vi "temp-control-tuner.vi"() -> ()   [LabVIEW 2013]
uses:
  <vilib>/Analysis/polynomials.llb/Scalar Polynomial Evaluation (DBL).vi
  <vilib>/Analysis/NI_AALPro.lvlib
panel:
  in  "Output Enable":bool
  in  "pwm_rate":dbl min=0.0 max=655.35
  in  "i_limit":u8
  in  "ki":dbl min=0.0 max=65.535
  in  "kp":dbl min=0.0 max=65.535
  in  "Write Tuning":bool
  in  "Temp Setpoint (degF)":dbl=32.0 min=32.0 max=1832.0 step=1.0
  out "Array":dbl[](array[numeric])
  in  "Write Setpoint":bool
  out "Waveform Chart":T1(graph)={"[0]"=63.3344, "[1]"=32.0, "[2]"=32.0, "[3]"=32.0, "[4]"=0.0, "[5]"=0.0, "[6]"=0.0, "[7]"=0.0, "[8]"=0.0}
  in  "stop":bool
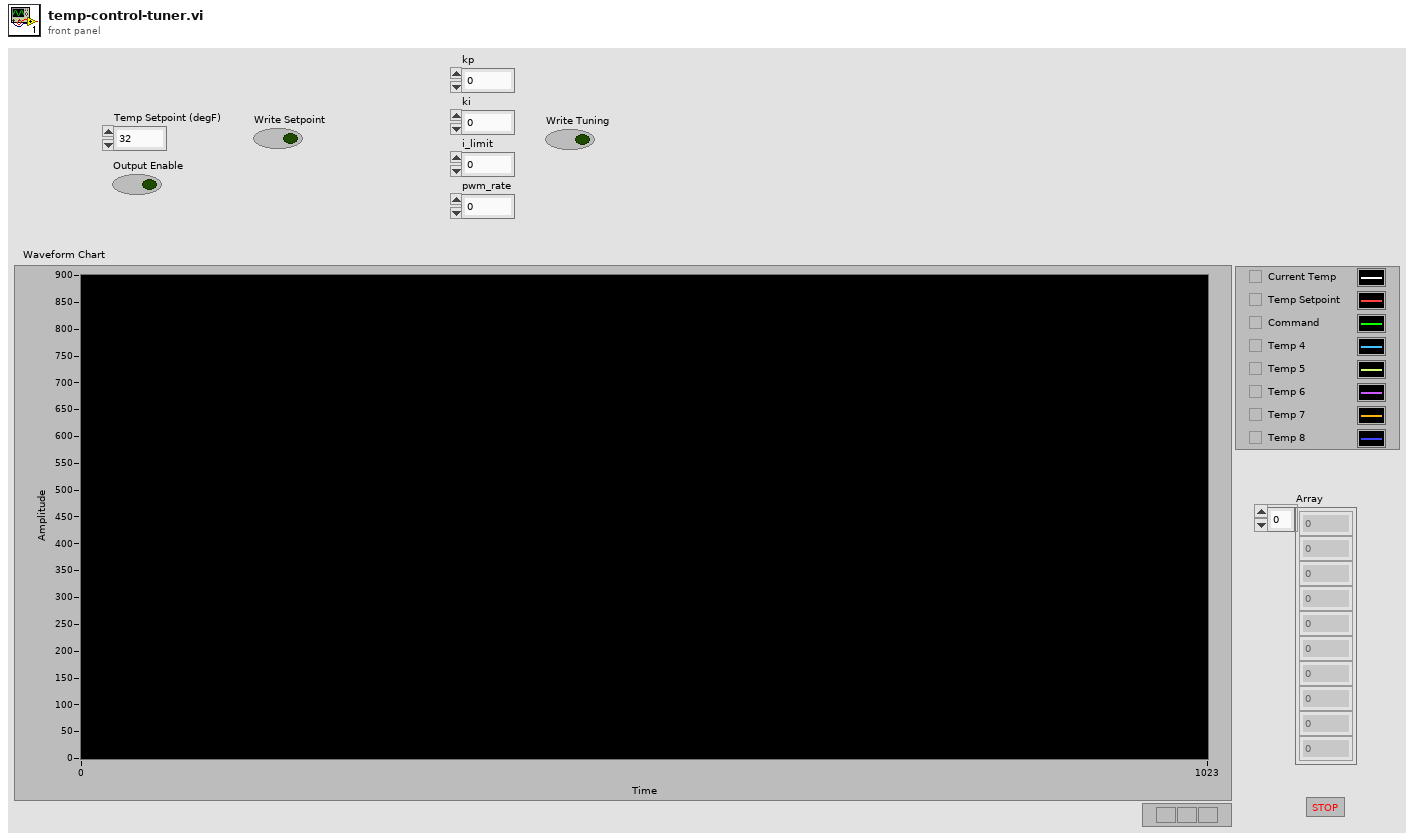
[diagram p1: front panel]
types:
  T1 = cluster{"[0]":dbl, "[1]":dbl, "[2]":dbl, "[3]":dbl, "[4]":dbl, "[5]":dbl, "[6]":dbl, "[7]":dbl, "[8]":dbl}
  T2 = enum16{"HSCAN", "MSCAN", "SWCAN", "LSFTCAN", "HSCAN2", "HSCAN3"}
  T3 = cluster{"DeviceType":i32, "Handle":i32, "NumberOfClients":i32, "SerialNumber":i32, "MaxAllowedClients":i32}[]
  T4 = cluster{"DeviceType":i32, "Handle":i32, "NumberOfClients":i32, "SerialNumber":i32, "MaxAllowedClients":i32}
  T5 = enum16{"DEVICE", "HSCAN", "MSCAN", "SWCAN", "LSFTCAN", "FORDSCP", "J1708", "JVPW", "ISO", "FIRE_HSCAN2", "FIRE_MSCAN1", "FIRE_HSCAN3", "FIRE_LIN2", "FIRE_LIN3", "FIRE_LIN4"}
  T6 = typedef "ctl spymessage.ctl" = cluster{"StatusBitField":u32, "StatusBitField2":u32, "TimeHardware":u32, "TimeHardware2":u32, "TimeSystem":u32, "TimeSystem2":u32, "TimeStampHardwareID":u8, "TimeStampHardwareID2":u8, "NetworkID":u8, "NodeID":u8, "Protocol":u8, "MessagePieceID":u8, "ColorID":u8, "NumberBytesHeader":u8, "NumberBytesData":u8, "DescriptionID":u16, "ArbIDOrHeader":u32, "Data [8]":u8[], "AckBytes [8]":u8[], "Value":sgl, "MiscData":u8}
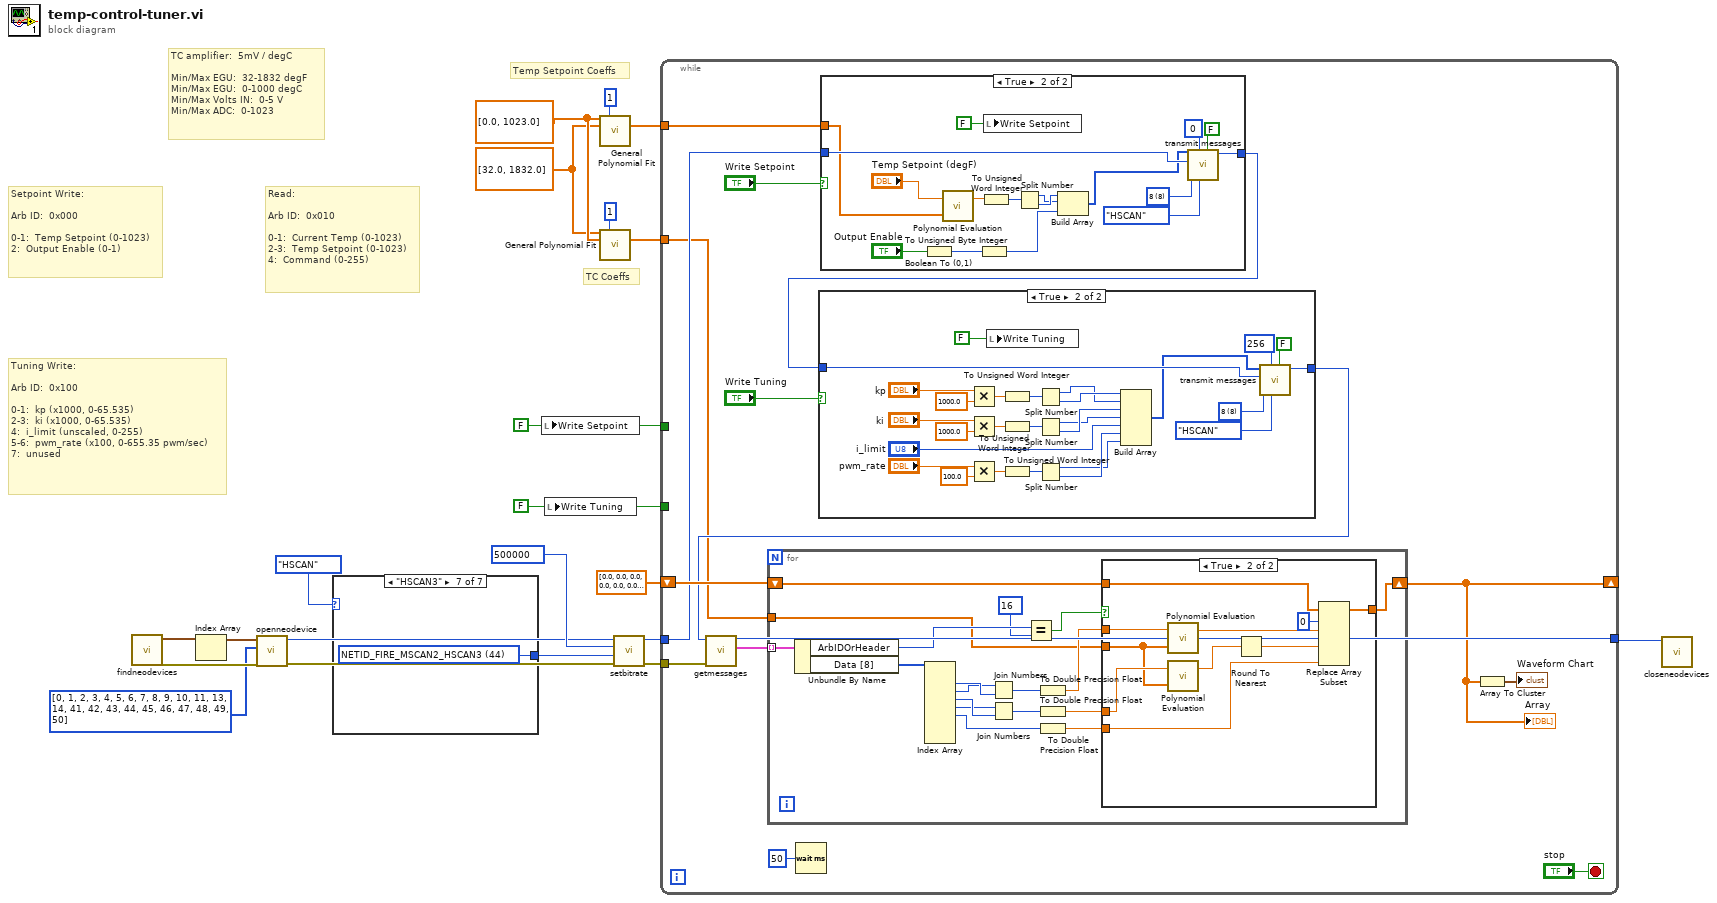
[diagram p0: block diagram]
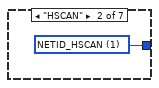
[diagram p3: hidden frame]
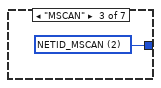
[diagram p4: hidden frame]
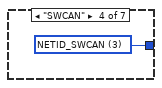
[diagram p5: hidden frame]
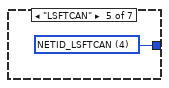
[diagram p6: hidden frame]
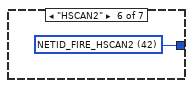
[diagram p7: hidden frame]
diagram:
  w5 = FALSE ("Send")
  w1 = dbl[] [32.0, 1832.0] ("Y")
  w2 = dbl[] [0.0, 1023.0] ("Y")
  w8 = FALSE ("Send")
  w15 = 500000 items=["20000"=20000, "33333"=33333, "50000"=50000, "62500"=62500, "83333"=83333, "100000"=100000, "125000"=125000, "250000"=250000, "500000"=500000, "800000"=800000, "1000000"=1000000] ("Bit Rate")
  w18 = i8[] [0, 1, 2, 3, 4, 5, 6, 7, 8, 9, 10, 11, 13, 14, 41, 42, 43, 44, 45, 46, 47, 48, 49, 50] items=["NETID_DEVICE"=0, "NETID_HSCAN"=1, "NETID_MSCAN"=2, "NETID_SWCAN"=3, "NETID_LSFTCAN"=4, "NETID_FORDSCP"=5, "NETID_J1708"=6, "NETID_AUX"=7, "NETID_JVPW"=8, "NETID_ISO_LIN"=9, "NETID_ISOPIC"=10, "NETID_MAIN51"=11, "NETID_SCI"=13, "NETID_ISO2"=14, "NETID_FIRE_HSCAN1"=41, "NETID_FIRE_HSCAN2"=42, "NETID_FIRE_MSCAN1"=43, "NETID_FIRE_MSCAN2_HSCAN3"=44, "NETID_FIRE_SWCAN"=45, "NETID_FIRE_LSFT"=46, "NETID_FIRE_LIN1"=47, "NETID_FIRE_LIN2"=48, "NETID_FIRE_LIN3"=49, "NETID_FIRE_LIN4"=50] ("bNetworkIDs")
  # "Temp Setpoint Coeffs"
  # "TC Coeffs"
  # "TC amplifier:  5mV / degC\n\nMin/Max EGU:  32-1832 degF\nMin/Max EGU:  0-1000 degC\nMin/Max Volts IN:  0-5 V\nMin/Max ADC:  0-1023"
  # "Read:\n\nArb ID:  0x010\n\n0-1:  Current Temp (0-1023)\n2-3:  Temp Setpoint (0-1023)\n4:  Command (0-255)"
  # "Tuning Write:\n\nArb ID:  0x100\n\n0-1:  kp (x1000, 0-65.535)\n2-3:  ki (x1000, 0-65.535)\n4:  i_limit (unscaled, 0-255)\n5-6:  pwm_rate (x100, 0-655.35 pwm/sec)\n7:  unused"
  # "Setpoint Write:\n\nArb ID:  0x000\n\n0-1:  Temp Setpoint (0-1023)\n2:  Output Enable (0-1)"
  n1 = call "findneodevices.vi"() -> ("error out"=w20:errorcluster, "NeoDevices {}"=w21:T3)  [unwired: 3 in, 7 out]
  n2 = Index Array(array=w21) -> (element=w19:T4)  [unwired: 1 in]
  n3 = call "openneodevice.vi"("error in (no error)"=w20, "bNetworkIDs"=w18, "NeoDevice{}"=w19) -> ("error out"=w12:errorcluster, "hObject"=w13:i32)  [unwired: 2 in, 5 out]
  n4 = case shown="\"HSCAN3\"" T2."HSCAN" ("CAN Channel") {
    tunnel: [_ w22 w23 w24 w25 w26 w27] -> w14
    frame Default {
    }
    frame "HSCAN" {
      w22 = i8 1 items=["NETID_DEVICE"=0, "NETID_HSCAN"=1, "NETID_MSCAN"=2, "NETID_SWCAN"=3, "NETID_LSFTCAN"=4, "NETID_FORDSCP"=5, "NETID_J1708"=6, "NETID_AUX"=7, "NETID_JVPW"=8, "NETID_ISO_LIN"=9, "NETID_ISOPIC"=10, "NETID_MAIN51"=11, "NETID_SCI"=13, "NETID_ISO2"=14, "NETID_FIRE_HSCAN1"=41, "NETID_FIRE_HSCAN2"=42, "NETID_FIRE_MSCAN1"=43, "NETID_FIRE_MSCAN2_HSCAN3"=44, "NETID_FIRE_SWCAN"=45, "NETID_FIRE_LSFT"=46, "NETID_FIRE_LIN1"=47, "NETID_FIRE_LIN2"=48, "NETID_FIRE_LIN3"=49, "NETID_FIRE_LIN4"=50] ("NetworkID")
    }
    frame "MSCAN" {
      w23 = i8 2 items=["NETID_DEVICE"=0, "NETID_HSCAN"=1, "NETID_MSCAN"=2, "NETID_SWCAN"=3, "NETID_LSFTCAN"=4, "NETID_FORDSCP"=5, "NETID_J1708"=6, "NETID_AUX"=7, "NETID_JVPW"=8, "NETID_ISO_LIN"=9, "NETID_ISOPIC"=10, "NETID_MAIN51"=11, "NETID_SCI"=13, "NETID_ISO2"=14, "NETID_FIRE_HSCAN1"=41, "NETID_FIRE_HSCAN2"=42, "NETID_FIRE_MSCAN1"=43, "NETID_FIRE_MSCAN2_HSCAN3"=44, "NETID_FIRE_SWCAN"=45, "NETID_FIRE_LSFT"=46, "NETID_FIRE_LIN1"=47, "NETID_FIRE_LIN2"=48, "NETID_FIRE_LIN3"=49, "NETID_FIRE_LIN4"=50] ("NetworkID")
    }
    frame "SWCAN" {
      w24 = i8 3 items=["NETID_DEVICE"=0, "NETID_HSCAN"=1, "NETID_MSCAN"=2, "NETID_SWCAN"=3, "NETID_LSFTCAN"=4, "NETID_FORDSCP"=5, "NETID_J1708"=6, "NETID_AUX"=7, "NETID_JVPW"=8, "NETID_ISO_LIN"=9, "NETID_ISOPIC"=10, "NETID_MAIN51"=11, "NETID_SCI"=13, "NETID_ISO2"=14, "NETID_FIRE_HSCAN1"=41, "NETID_FIRE_HSCAN2"=42, "NETID_FIRE_MSCAN1"=43, "NETID_FIRE_MSCAN2_HSCAN3"=44, "NETID_FIRE_SWCAN"=45, "NETID_FIRE_LSFT"=46, "NETID_FIRE_LIN1"=47, "NETID_FIRE_LIN2"=48, "NETID_FIRE_LIN3"=49, "NETID_FIRE_LIN4"=50] ("NetworkID")
    }
    frame "LSFTCAN" {
      w25 = i8 4 items=["NETID_DEVICE"=0, "NETID_HSCAN"=1, "NETID_MSCAN"=2, "NETID_SWCAN"=3, "NETID_LSFTCAN"=4, "NETID_FORDSCP"=5, "NETID_J1708"=6, "NETID_AUX"=7, "NETID_JVPW"=8, "NETID_ISO_LIN"=9, "NETID_ISOPIC"=10, "NETID_MAIN51"=11, "NETID_SCI"=13, "NETID_ISO2"=14, "NETID_FIRE_HSCAN1"=41, "NETID_FIRE_HSCAN2"=42, "NETID_FIRE_MSCAN1"=43, "NETID_FIRE_MSCAN2_HSCAN3"=44, "NETID_FIRE_SWCAN"=45, "NETID_FIRE_LSFT"=46, "NETID_FIRE_LIN1"=47, "NETID_FIRE_LIN2"=48, "NETID_FIRE_LIN3"=49, "NETID_FIRE_LIN4"=50] ("NetworkID")
    }
    frame "HSCAN2" {
      w26 = i8 42 items=["NETID_DEVICE"=0, "NETID_HSCAN"=1, "NETID_MSCAN"=2, "NETID_SWCAN"=3, "NETID_LSFTCAN"=4, "NETID_FORDSCP"=5, "NETID_J1708"=6, "NETID_AUX"=7, "NETID_JVPW"=8, "NETID_ISO_LIN"=9, "NETID_ISOPIC"=10, "NETID_MAIN51"=11, "NETID_SCI"=13, "NETID_ISO2"=14, "NETID_FIRE_HSCAN1"=41, "NETID_FIRE_HSCAN2"=42, "NETID_FIRE_MSCAN1"=43, "NETID_FIRE_MSCAN2_HSCAN3"=44, "NETID_FIRE_SWCAN"=45, "NETID_FIRE_LSFT"=46, "NETID_FIRE_LIN1"=47, "NETID_FIRE_LIN2"=48, "NETID_FIRE_LIN3"=49, "NETID_FIRE_LIN4"=50] ("NetworkID")
    }
    frame "HSCAN3" {
      w27 = i8 44 items=["NETID_DEVICE"=0, "NETID_HSCAN"=1, "NETID_MSCAN"=2, "NETID_SWCAN"=3, "NETID_LSFTCAN"=4, "NETID_FORDSCP"=5, "NETID_J1708"=6, "NETID_AUX"=7, "NETID_JVPW"=8, "NETID_ISO_LIN"=9, "NETID_ISOPIC"=10, "NETID_MAIN51"=11, "NETID_SCI"=13, "NETID_ISO2"=14, "NETID_FIRE_HSCAN1"=41, "NETID_FIRE_HSCAN2"=42, "NETID_FIRE_MSCAN1"=43, "NETID_FIRE_MSCAN2_HSCAN3"=44, "NETID_FIRE_SWCAN"=45, "NETID_FIRE_LSFT"=46, "NETID_FIRE_LIN1"=47, "NETID_FIRE_LIN2"=48, "NETID_FIRE_LIN3"=49, "NETID_FIRE_LIN4"=50] ("NetworkID")
    }
  }
  n5 = local write "Write Setpoint"(w8) -> ()
  n6 = local write "Write Tuning"(w5) -> ()
  n7 = call <vilib>:"General Polynomial Fit.vi"("Y"=w2, "polynomial order"=1, "X"=w1) -> ("Polynomial Coefficients"=w3:dbl[])  [unwired: 9 in, 3 out]
  n8 = call <vilib>:"General Polynomial Fit.vi"("Y"=w1, "polynomial order"=1, "X"=w2) -> ("Polynomial Coefficients"=w4:dbl[])  [unwired: 9 in, 3 out]
  n9 = call "setbitrate.vi"("error in (no error)"=w12, "NetworkID"=w14, "BitRate"=w15, "hObject"=w13) -> ("error out"=w10:errorcluster, "hObject Out"=w11:i32)  [unwired: 6 out]
  n10 = while {
    tunnel: w11 -> [w34]
    tunnel: w10 -> [w41]
    tunnel: [w38] -> w17
    shift-right: [w35] -> _
    shift-left: dbl[] [0.0, 0.0, 0.0, 0.0, 0.0, 0.0, 0.0, 0.0] -> [w37]
    tunnel: w8 -> [_]
    tunnel: w5 -> [_]
    tunnel: w4 -> [w29]
    tunnel: w3 -> [w28]
    stop <- "stop" stop-if-true
    n11 = Wait (ms)(milliseconds to wait=u32 50) -> ()  [unwired: 1 out]
    n12 = case shown="True" "Write Setpoint" {
      tunnel: w34 -> [w71 w84]
      tunnel: [w71 w82] -> w31
      tunnel: w28 -> [_ w81]
      frame False {
      }
      frame True {
        w86 = 8 items=["0", "1", "2", "3", "4", "5", "6", "7", "8", "9", "10", "11"] ("Number of \nData Bytes")
        n13 = Boolean To (0,1)(Boolean="Output Enable") -> (0, 1=w73:i16)
        n14 = call-poly <vilib>:"Polynomial Evaluation.vi"("P(x)"=w81, "a"="Temp Setpoint (degF)") -> ("P(a)"=w79:dbl)  [unwired: 1 out]
        n15 = To Unsigned Byte Integer(number=w73) -> (unsigned 8bit integer=w72:u8)
        n16 = To Unsigned Word Integer(number=w79) -> (unsigned 16bit integer=w77:u16)
        n17 = local write "Write Setpoint"(FALSE ("Send")) -> ()
        n18 = Split Number(x=w77) -> (hi(x)=w75:u8, lo(x)=w76:u8)
        n19 = Build Array(w76, w75, w72) -> (w78:u8[])
        n20 = call "transmit messages.vi"("extended ID?"=FALSE ("Send Extended ID"), "Network"=T5."HSCAN", "Arb ID"=u32 0, "Number of \nData Bytes"=w86, "hObject In"=w84, "Data"=w78) -> ("hObject Out"=w82:i32)  [unwired: 1 in, 4 out]
      }
    }
    n21 = case shown="True" "Write Tuning" {
      tunnel: w31 -> [w43 w66]
      tunnel: [w43 w64] -> w30
      frame False {
      }
      frame True {
        w68 = 8 items=["0", "1", "2", "3", "4", "5", "6", "7", "8", "9", "10", "11"] ("Number of \nData Bytes")
        n22 = Multiply(x="kp", y=1000.0) -> (x*y=w56:dbl)
        n23 = Multiply(x="ki", y=1000.0) -> (x*y=w54:dbl)
        n24 = Multiply(x="pwm_rate", y=100.0) -> (x*y=w52:dbl)
        n25 = local write "Write Tuning"(FALSE ("Send")) -> ()
        n26 = To Unsigned Word Integer(number=w56) -> (unsigned 16bit integer=w57:u16)
        n27 = To Unsigned Word Integer(number=w54) -> (unsigned 16bit integer=w55:u16)
        n28 = To Unsigned Word Integer(number=w52) -> (unsigned 16bit integer=w53:u16)
        n29 = Split Number(x=w57) -> (hi(x)=w50:u8, lo(x)=w51:u8)
        n30 = Split Number(x=w55) -> (hi(x)=w48:u8, lo(x)=w49:u8)
        n31 = Split Number(x=w53) -> (hi(x)=w45:u8, lo(x)=w46:u8)
        n32 = Build Array(w51, w50, w49, w48, "i_limit", w46, w45) -> (w44:u8[])
        n33 = call "transmit messages.vi"("extended ID?"=FALSE ("Send Extended ID"), "Network"=T5."HSCAN", "Arb ID"=u32 256, "Number of \nData Bytes"=w68, "hObject In"=w66, "Data"=w44) -> ("hObject Out"=w64:i32)  [unwired: 1 in, 4 out]
      }
    }
    n34 = call "getmessages.vi"("error in (no error)"=w41, "hObject"=w30) -> ("pMsgs"=w42:T6[], "hObject Out"=w38:i32)  [unwired: 8 out]
    n35 = for {
      tunnel: w42 -> [w106] mode=indexing
      shift-right: [w100] -> w35
      shift-left: w37 -> [w102]
      tunnel: w29 -> [w90]
      n36 = Unbundle By Name(w106) -> ("ArbIDOrHeader"=w99:u32, "Data [8]"=w105:u8[])
      n37 = Index Array(array=w105) -> (element #1=w104:u8, element #2=w103:u8, element #3=w94:u8, element #4=w93:u8, element #5=w92:u8)  [unwired: 8 in, 3 out]
      n38 = Join Numbers(hi=w103, lo=w104) -> ((hi.lo)=w97:u16)
      n39 = Join Numbers(hi=w93, lo=w94) -> ((hi.lo)=w95:u16)
      n40 = Equal?(x=w99, y=u32 16 ("Arb ID")) -> (x = y?=w98:bool)
      n41 = To Double Precision Float(number=w97) -> (double precision float=w101:dbl)
      n42 = To Double Precision Float(number=w95) -> (double precision float=w91:dbl)
      n43 = To Double Precision Float(number=w92) -> (double precision float=w89:dbl)
      n44 = case shown="True" w98 {
        tunnel: w102 -> [w107 w117]
        tunnel: w101 -> [_ w114]
        tunnel: [w107 w116] -> w100
        tunnel: w91 -> [_ w113]
        tunnel: w90 -> [_ w112]
        tunnel: w89 -> [_ w109]
        frame False {
        }
        frame True {
          n45 = call-poly <vilib>:"Polynomial Evaluation.vi"("P(x)"=w112, "a"=w114) -> ("P(a)"=w111:dbl)  [unwired: 1 out]
          n46 = call-poly <vilib>:"Polynomial Evaluation.vi"("P(x)"=w112, "a"=w113) -> ("P(a)"=w110:dbl)  [unwired: 1 out]
          n47 = Round To Nearest(number=w110) -> (nearest integer value=w108:dbl)
          n48 = Replace Array Subset(array=w117, new element #1=w111, index #1=0 ("index"), new element #2=w108, new element #3=w109) -> (w116:dbl[])  [unwired: 2 in]
        }
      }
    }
    "Array" <- w35
    n49 = Array To Cluster(array=w35) -> (cluster=→"Waveform Chart":T1)
  }
  n50 = call "closeneodevices.vi"("hObject"=w17) -> ()  [unwired: 2 in, 9 out]
